vi "Init.vi"(0 "Physical Channel":tag="TS1Mod1/power", 11 "error in (no error)":errorcluster) -> (4 "task out":refnum<k21>, 15 "error out":errorcluster)   [LabVIEW 2021, in "Z Power Module Power Measurement.lvlib"]
doc: "This VI creates a task for the selected Physical channel"
uses:
  Z Power Module Power Measurement.lvlib
  <vilib>/DAQmx/create/channels.llb/DAQmx Create Channel (Power).vi
panel:
  # "INPUT"
  # "OUTPUT"
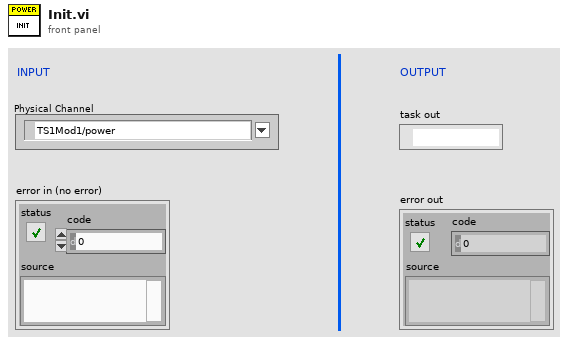
[diagram p1: front panel]
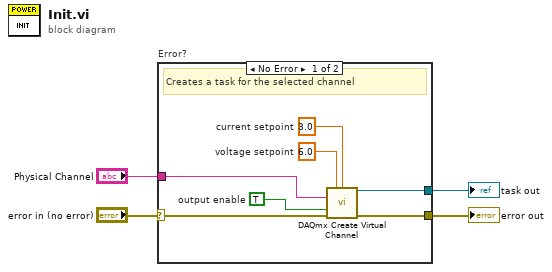
[diagram p0: block diagram]
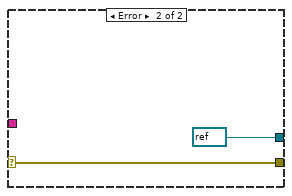
[diagram p2: hidden frame]
diagram:
  n1 = case "Error?" shown="No Error" "error in (no error)" {
    selector: "error in (no error)" -> [w11 w13]
    tunnel: [w10 refnum<k21> refnum ("task out")] -> w3
    tunnel: [w8 w13] -> w2
    tunnel: "Physical Channel" -> [w7 _]
    frame No Error {
      w5 = 6.0  # voltage setpoint
      w6 = 3.0  # current setpoint
      w9 = TRUE  # output enable
      # "Creates a task for the selected channel"
      n2 = call-poly <vilib>:"DAQmx Create Virtual Channel.vi"("voltage setpoint"=w5, "current setpoint"=w6, "physical channels"=w7, "output enable"=w9, "error in"=w11) -> ("task out"=w10:refnum<k21>, "error out"=w8:errorcluster)  [unwired: 9 in]
    }
    frame Error {
    }
  }
  "error out" <- w2
  "task out" <- w3
